vi "Check Items for Modifications.vi"(9 "Saved Item Data":refnum<class "Item.lvclass">[](array[class]), 11 "New Item Data":refnum<class "Item.lvclass">[](array[class])) -> (1 "Number of Modified Items":i32, 3 "New Item Data w/ Mod Bit Set":refnum<class "Item.lvclass">[](array[class]))   [LabVIEW 2020, in "VI Properties Editor.lvlib"]
doc: "Checks each item to see if modifications have been made, and sets an internal modification bit to TRUE if so."
uses:
  VI Properties Editor.lvlib
  Classes/Item/Item.lvclass
  <vilib>/LabVIEW Icon API/lv_icon/Classes/Icon/Icon.lvclass
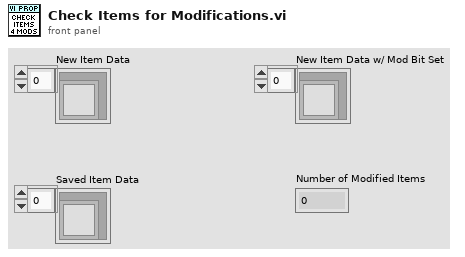
[diagram p1: front panel]
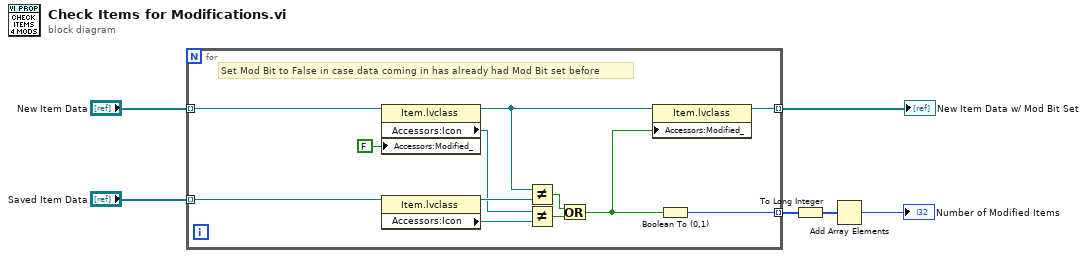
[diagram p0: block diagram]
diagram:
  n1 = for {
    tunnel: "Saved Item Data" -> [w17] mode=indexing
    tunnel: "New Item Data" -> [w8] mode=indexing
    tunnel: [w18] -> w1 mode=indexing
    tunnel: [w11] -> w4 mode=indexing
    # "Set Mod Bit to False in case data coming in has already had Mod Bit set before"
    n2 = property class="Item.lvclass"(reference=w8, "Accessors:Modified_"=FALSE ("Modified?")) -> (reference out=w10:refnum<class "Item.lvclass">, "Accessors:Icon"=w15:refnum<class "Icon.lvclass">)  [unwired: 1 in, 1 out]
    n3 = property class="Item.lvclass"(reference=w17) -> (reference out=w16:refnum<class "Item.lvclass">, "Accessors:Icon"=w14:refnum<class "Icon.lvclass">)  [unwired: 1 in, 1 out]
    n4 = Not Equal?(x=w10, y=w16) -> (x != y?=w12:bool)
    n5 = Not Equal?(x=w15, y=w14) -> (x != y?=w13:bool)
    n6 = Or(x=w12, y=w13) -> (x .or. y?=w9:bool)
    n7 = property class="Item.lvclass"(reference=w10, "Accessors:Modified_"=w9) -> (reference out=w18:refnum<class "Item.lvclass">)  [unwired: 1 in, 1 out]
    n8 = Boolean To (0,1)(Boolean=w9) -> (0, 1=w11:i16)
  }
  "New Item Data w/ Mod Bit Set" <- w1
  n9 = To Long Integer(number=w4) -> (32bit integer=w2:i32[])
  n10 = Add Array Elements(numeric array=w2) -> (sum=→"Number of Modified Items":i32)
